vi "GERG04dll.vi"(8 "error in (no error)":errorcluster, 11 "Inputs":cluster{"ncc":i32, "iflag":i32}) -> (0 "error out":errorcluster, 3 "Outputs":T1)   [LabVIEW 2015]
doc: "subroutine GERG04dll(ncc, iflag, ierr, herr, herr_length)\n\nset the pure model(s) to those used by the GERG 2004 formulation.\n\nThis subroutine must be called before SETUP; it need not be called\nat all if the default (NIST-recommended) models are desired.\n\nTo turn off the GERG settings, call this routine again with iflag=0,\nand then call the SETUP routine to reset the parameters of the equations\nof state.\n\nINPUTS:\nncc -- number of components (1 for pure fluid)\niflag -- set to 1 to load the GERG 2004 equations, set to 0 for defaults\n\nOUTPUTS:\nierr -- error flag: 0 = successful\nherr -- error string returned from SETMOD\nherr_length -- length of variable herr (default: 255)"
uses:
  REFPROP.dll
panel:
  # "REFPROP-GERG04dll.vi"
  # "void  GERG04dll(int32_t *ncc, int32_t *iflag, int32_t *ierr, CStr herr, int32_t herr_length);"
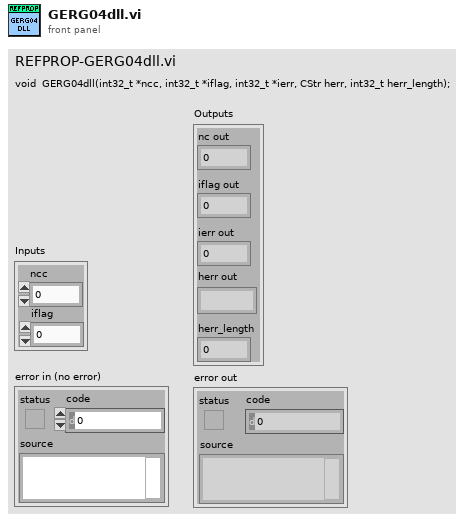
[diagram p1: front panel]
types:
  T1 = cluster{"nc out":i32, "iflag out":i32, "ierr out":i32, "herr out":string, "herr_length":i32}
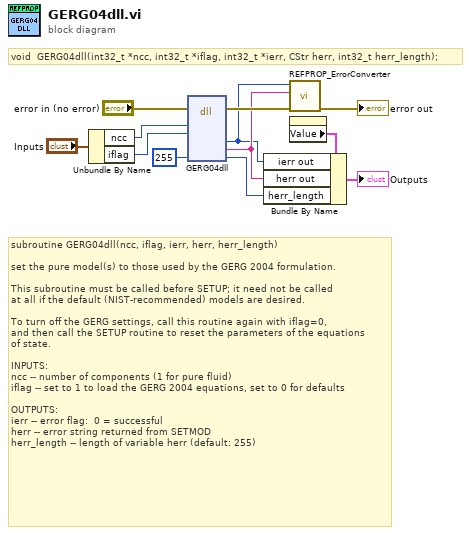
[diagram p0: block diagram]
diagram:
  # "void  GERG04dll(int32_t *ncc, int32_t *iflag, int32_t *ierr, CStr herr, int32_t herr_length);"
  # "subroutine GERG04dll(ncc, iflag, ierr, herr, herr_length)\n\nset the pure model(s) to those used by the GERG 2004 formulation.\n\nThis subroutine must be called before SETUP; it need not be called\nat all if the default (NIST-recommended) models are desired.\n\nTo turn off the GERG settings, call this routine again with iflag=0,\nand then call the SETUP routine to reset the parameters of the equations\nof state.\n\nINPUTS:\nncc -- number of components (1 for pure fluid)\niflag -- set to 1 to load the GERG 2004 equations, set to 0 for defaults\n\nOUTPUTS:\nierr -- error flag:  0 = successful\nherr -- error string returned from SETMOD\nherr_length -- length of variable herr (default: 255)"
  n1 = Unbundle By Name("Inputs") -> ("ncc"=w4:i32, "iflag"=w3:i32)
  n2 = dll-call lib="C:/Users/lauria/Desktop/REFPROP 10 LabVIEW Wrapper BETA/REFPROP/REFPROP.*" fn="GERG04dll"(error in="error in (no error)", "ncc"=w4, "iflag"=w3, "herr_length"=255) -> (error out=w12:errorcluster, "ierr"=w1:i32, "herr"=w2:string, "herr_length"=w7:i32)  [unwired: 7 in, 1 out]
  n3 = call "REFPROP_ErrorConverter.vi"("error in (no error)"=w12, "Error Message"=w2, "Error Code"=w1) -> ("error out"=→"error out":errorcluster)  [unwired: 8 in]
  n4 = property on="Outputs" class="Clust (strict)"() -> ("Value"=w8:T1)  [unwired: 2 in, 2 out]
  n5 = Bundle By Name(cluster=w8, "ierr out"=w1, "herr out"=w2, "herr_length"=w7) -> (→"Outputs":T1)
